vi "メイン.vi"() -> (2 "測定周期/ms":dbl, 3 "値転記用配列":T2[](array[typedef]))   [LabVIEW 2021] (continued)
        n1474 = local read "メイン設定_設定 6"() -> (w3404:T2)
        n1475 = Bundle By Name(cluster=w3404, "実測値(MAX)"=w3400, "実測値(MIN)"=w3400) -> (w3403:T2)
        n1476 = local write "メイン設定_設定 6"(w3403) -> ()
        n1477 = global write "測定値MAXMIN_G.vi" "測定値MAX/MINグローバル"(string[][] []) -> ()
      }
      frame "値7クリア" {
        w3405 = ""
        # "測定値MAX/MINグローバルの値を初期化する"
        # "②"
        # "①"
        # "複製したら変更する項目\n①②\nローカル変数\n\n変更のみでOK"
        # "項目別の値のクリアの為、項目配列の分だけ作成する"
        n1478 = local read "メイン設定_設定 7"() -> (w3409:T2)
        n1479 = Bundle By Name(cluster=w3409, "実測値(MAX)"=w3405, "実測値(MIN)"=w3405) -> (w3408:T2)
        n1480 = local write "メイン設定_設定 7"(w3408) -> ()
        n1481 = global write "測定値MAXMIN_G.vi" "測定値MAX/MINグローバル"(string[][] []) -> ()
      }
      frame "値8クリア" {
        w3410 = ""
        # "測定値MAX/MINグローバルの値を初期化する"
        # "②"
        # "①"
        # "複製したら変更する項目\n①②\nローカル変数\n\n変更のみでOK"
        # "項目別の値のクリアの為、項目配列の分だけ作成する"
        n1482 = local read "メイン設定_設定 8"() -> (w3414:T2)
        n1483 = Bundle By Name(cluster=w3414, "実測値(MAX)"=w3410, "実測値(MIN)"=w3410) -> (w3413:T2)
        n1484 = local write "メイン設定_設定 8"(w3413) -> ()
        n1485 = global write "測定値MAXMIN_G.vi" "測定値MAX/MINグローバル"(string[][] []) -> ()
      }
      frame "値9クリア" {
        w3415 = ""
        # "測定値MAX/MINグローバルの値を初期化する"
        # "②"
        # "①"
        # "複製したら変更する項目\n①②\nローカル変数\n\n変更のみでOK"
        # "項目別の値のクリアの為、項目配列の分だけ作成する"
        n1486 = local read "メイン設定_設定 9"() -> (w3419:T2)
        n1487 = Bundle By Name(cluster=w3419, "実測値(MAX)"=w3415, "実測値(MIN)"=w3415) -> (w3418:T2)
        n1488 = local write "メイン設定_設定 9"(w3418) -> ()
        n1489 = global write "測定値MAXMIN_G.vi" "測定値MAX/MINグローバル"(string[][] []) -> ()
      }
      frame "値10クリア" {
        w3420 = ""
        # "測定値MAX/MINグローバルの値を初期化する"
        # "②"
        # "①"
        # "複製したら変更する項目\n①②\nローカル変数\n\n変更のみでOK"
        # "項目別の値のクリアの為、項目配列の分だけ作成する"
        n1490 = local read "メイン設定_設定 10"() -> (w3424:T2)
        n1491 = Bundle By Name(cluster=w3424, "実測値(MAX)"=w3420, "実測値(MIN)"=w3420) -> (w3423:T2)
        n1492 = local write "メイン設定_設定 10"(w3423) -> ()
        n1493 = global write "測定値MAXMIN_G.vi" "測定値MAX/MINグローバル"(string[][] []) -> ()
      }
      frame "値11クリア" {
        w3425 = ""
        # "測定値MAX/MINグローバルの値を初期化する"
        # "②"
        # "①"
        # "複製したら変更する項目\n①②\nローカル変数\n\n変更のみでOK"
        # "項目別の値のクリアの為、項目配列の分だけ作成する"
        n1494 = local read "メイン設定_設定 11"() -> (w3429:T2)
        n1495 = Bundle By Name(cluster=w3429, "実測値(MAX)"=w3425, "実測値(MIN)"=w3425) -> (w3428:T2)
        n1496 = local write "メイン設定_設定 11"(w3428) -> ()
        n1497 = global write "測定値MAXMIN_G.vi" "測定値MAX/MINグローバル"(string[][] []) -> ()
      }
      frame "値12クリア" {
        w3430 = ""
        # "測定値MAX/MINグローバルの値を初期化する"
        # "②"
        # "①"
        # "複製したら変更する項目\n①②\nローカル変数\n\n変更のみでOK"
        # "項目別の値のクリアの為、項目配列の分だけ作成する"
        n1498 = local read "メイン設定_設定 12"() -> (w3434:T2)
        n1499 = Bundle By Name(cluster=w3434, "実測値(MAX)"=w3430, "実測値(MIN)"=w3430) -> (w3433:T2)
        n1500 = local write "メイン設定_設定 12"(w3433) -> ()
        n1501 = global write "測定値MAXMIN_G.vi" "測定値MAX/MINグローバル"(string[][] []) -> ()
      }
      frame "測定1" {
        # "項目別のボタンで測定を行う為、項目分必要"
        n1502 = local read "測定旧値 1"() -> (w3437:bool)
        n1503 = case shown="FALSE" w3437 {
          tunnel: w3435 -> [w3440 w3703]
          tunnel: [w3439 w3703] -> w3436
          frame False {
            n1504 = flat-sequence {
              tunnel: w3440 -> [w3450]
              tunnel: [w3441] -> w3438
              tunnel: [w3688] -> w3439
              tunnel: w3438 -> [w3688]
              frame #0 {
                # "※複製コピー時変更する項目\n①②\nローカル変数\n\n入れ子のケースストラクチャ\"2\"を複製\n\n0～数だけ変更する\n③④⑤\nローカル変数\n\n※AB\n行番号の変更をする必要がある\n\n--------------------------------\nこの後イベントストラクチャ複製する\n--------------------------------\nイベントストラクチャ複製後\n\n⑦⑧\nローカル変数\n⑨\n装飾体の位置設定\n-51は固定\n前ケースの数値+72\n⑩\n測定新値リセット用\nのボタンが複製されているので、\nフロントパネルを整理する\n⑪\nプロパティノード\nボタンの無効解除クリア以外全てのボタン対象"
                # "実測完了\n1)測定モードが単発・連続、多点かで転記する配列を変える\n2)値転記用配列へ転記\n\nここからゲージ分を繰り返す必要がある\n\n3)配列0を取り出す\n4)配列0のポートNoを取り出す\n5)メイン測定_設定配列(測定1の対象配列)のポートNoと比較\n6)同じだったら処理をする。違ったら何もしない\n7)同じだったら配列0のメインON/OFF_設定1の使用ON/OFFがTrueかFalseか\nFlaseだったら前回値転記用配列から前回の値をメイン設定_設定へ転記\nTrueだったらメイン設定_設定の測定モードから\n0単発、1連続、3多点\nの処理を行う\n8)測定値をメイン設定_設定へ転記したら、前回転記用配列へ転記する"
                # "グループNO(表示上はポートNo)が同じだったら値を転記する\n\n測定した配列のグループNOと値転記用配列の他の指標グループNOを比較する\n＝だったら、対象の配列のON/OFFボタンがTrueか確認し、\nTrueだったら、測定モードによって、値かMAX、MINの数値を転記する\n\nグループNOが同じでなければ、転記しない(何もしない)"
                # "まず値転記用配列に測定の値を転記"
                # "設定項目の値へ値転記用配列から転記\n測定モードによって転記の値をMAXのみするか\nMAXとMINにするか分ける"
                # "実測定画面vi動作"
                n1505 = local read "メイン設定_設定 1"() -> (w3447:T2)
                n1506 = local read "測定周期/ms"() -> (w3448:dbl)
                n1507 = local read "測定新値 1"() -> (→"測定新値\nリセット用 1":bool)
                n1508 = Unbundle By Name(w3447) -> ("測定モード"=w3446:u16)
                n1509 = call "実測定画面.vi"("実測設定項目配列_\nメインからの転記"=w3450, "測定周期/ms_制御器"=w3448) -> ("実測設定項目配列_\nゲージIOへ転記用"=w3445:T2[], "実測設定項目配列_\n多点測定メイン転記用"=w3444:T2[])  [unwired: 11 in, 1 out]
                n1510 = case shown="2" w3446 {
                  tunnel: w3445 -> [w3457 w3458 _]
                  tunnel: [w3457 w3458 w3459] -> w3442
                  tunnel: w3444 -> [_ _ w3459]
                  frame 0, Default {
                  }
                  frame 1 {
                  }
                  frame 2 {
                  }
                }
                n1511 = for {
                  N: 32 -> [_]
                  tunnel: w3442 -> [w3466]
                  i -> [w3461]
                  # "32回分"
                  # "比較する固定GNO"
                  n1512 = local read "メイン設定_設定 1"() -> (w3460:T2)
                  n1513 = Index Array(array=w3466, index=w3461) -> (element=w3465:T2)
                  n1514 = Unbundle By Name(w3465) -> ("ポートNo."=w3463:dbl)
                  n1515 = Unbundle By Name(w3460) -> ("ポートNo."=w3464:dbl)
                  n1516 = Equal?(x=w3464, y=w3463) -> (x = y?=w3462:bool)
                  n1517 = case shown="TRUE" w3462 {
                    tunnel: w3465 -> [_ w3468]
                    tunnel: w3461 -> [_ w3467]
                    frame False {
                    }
                    frame True {
                      n1518 = case shown="0, デフォルト" w3467 {
                        tunnel: w3468 -> [w3484 w3502 w3520 w3538 w3556 w3574 w3592 w3610 w3628 w3646 w3664 w3682]
                        tunnel: w3467 -> [w3483 w3501 w3519 w3537 w3555 w3573 w3591 w3609 w3627 w3645 w3663 w3681]
                        frame 0, Default {
                          w3474 = 2
                          # "B"
                          # "A"
                          # "csv作成の為表へクラスタ(実測値)書き込み"
                          # "⑤"
                          # "③"
                          # "④"
                          n1519 = local read "メインON/OFF_\n設定 1"() -> (w3485:T1)
                          n1520 = Unbundle By Name(w3485) -> ("使用ON/OFF"=w3481:bool)
                          n1521 = control-ref of="前回値転記用配列"() -> (w3479:refnum<vi>)
                          n1522 = local read "メイン設定_設定 1"() -> (w3486:T2)
                          n1523 = call "メイン_測定値配列_CSV転記サブ.vi"("メイン設定_設定入力"=w3486, "ループ反復数値入力"=w3483, "実測設定項目"=w3484, "使用ON/OFF"=w3481, "前回値転記用配列"=w3479) -> ("ループ反復数値出力"=w3482:i32, "メイン設定_設定出力"=w3480:T2)  [unwired: 5 in]
                          n1524 = local write "メイン設定_設定 1"(w3480) -> ()
                          n1525 = Add(x=2, y=w3482) -> (x+y=w3475:i32)
                          n1526 = Add(x=w3482, y=3) -> (x+y=w3473:i32)
                          n1527 = local read "csv作成表"() -> (w3469:string[][])
                          n1528 = Unbundle By Name(w3480) -> ("実測値(MAX)"=w3476:string, "実測値(MIN)"=w3477:string)
                          n1529 = Replace Array Subset(array=w3469, new element #1=w3476, index (row) #1=w3474, index (col) #1=w3475, new element #2=w3477, index (row) #2=w3474, index (col) #2=w3473) -> (w3471:string[][])
                          n1530 = Select(t=w3471, s=w3481, f=w3469) -> (s? t:f=w3472:string[][])
                          n1531 = local write "csv作成表"(w3472) -> ()
                        }
                        frame 1 {
                          w3492 = 2
                          # "B"
                          # "A"
                          # "csv作成の為表へクラスタ(実測値)書き込み"
                          # "⑤"
                          # "③"
                          # "④"
                          n1532 = local read "メインON/OFF_\n設定 2"() -> (w3503:T1)
                          n1533 = Unbundle By Name(w3503) -> ("使用ON/OFF"=w3499:bool)
                          n1534 = control-ref of="前回値転記用配列"() -> (w3497:refnum<vi>)
                          n1535 = local read "メイン設定_設定 2"() -> (w3504:T2)
                          n1536 = call "メイン_測定値配列_CSV転記サブ.vi"("メイン設定_設定入力"=w3504, "ループ反復数値入力"=w3501, "実測設定項目"=w3502, "使用ON/OFF"=w3499, "前回値転記用配列"=w3497) -> ("ループ反復数値出力"=w3500:i32, "メイン設定_設定出力"=w3498:T2)  [unwired: 5 in]
                          n1537 = local write "メイン設定_設定 2"(w3498) -> ()
                          n1538 = Add(x=3, y=w3500) -> (x+y=w3493:i32)
                          n1539 = Add(x=w3500, y=4) -> (x+y=w3491:i32)
                          n1540 = local read "csv作成表"() -> (w3487:string[][])
                          n1541 = Unbundle By Name(w3498) -> ("実測値(MAX)"=w3494:string, "実測値(MIN)"=w3495:string)
                          n1542 = Replace Array Subset(array=w3487, new element #1=w3494, index (row) #1=w3492, index (col) #1=w3493, new element #2=w3495, index (row) #2=w3492, index (col) #2=w3491) -> (w3489:string[][])
                          n1543 = Select(t=w3489, s=w3499, f=w3487) -> (s? t:f=w3490:string[][])
                          n1544 = local write "csv作成表"(w3490) -> ()
                        }
                        frame 2 {
                          w3510 = 2
                          # "B"
                          # "A"
                          # "csv作成の為表へクラスタ(実測値)書き込み"
                          # "⑤"
                          # "③"
                          # "④"
                          n1545 = local read "メインON/OFF_\n設定 3"() -> (w3521:T1)
                          n1546 = Unbundle By Name(w3521) -> ("使用ON/OFF"=w3517:bool)
                          n1547 = control-ref of="前回値転記用配列"() -> (w3515:refnum<vi>)
                          n1548 = local read "メイン設定_設定 3"() -> (w3522:T2)
                          n1549 = call "メイン_測定値配列_CSV転記サブ.vi"("メイン設定_設定入力"=w3522, "ループ反復数値入力"=w3519, "実測設定項目"=w3520, "使用ON/OFF"=w3517, "前回値転記用配列"=w3515) -> ("ループ反復数値出力"=w3518:i32, "メイン設定_設定出力"=w3516:T2)  [unwired: 5 in]
                          n1550 = local write "メイン設定_設定 3"(w3516) -> ()
                          n1551 = Add(x=4, y=w3518) -> (x+y=w3511:i32)
                          n1552 = Add(x=w3518, y=5) -> (x+y=w3509:i32)
                          n1553 = local read "csv作成表"() -> (w3505:string[][])
                          n1554 = Unbundle By Name(w3516) -> ("実測値(MAX)"=w3512:string, "実測値(MIN)"=w3513:string)
                          n1555 = Replace Array Subset(array=w3505, new element #1=w3512, index (row) #1=w3510, index (col) #1=w3511, new element #2=w3513, index (row) #2=w3510, index (col) #2=w3509) -> (w3507:string[][])
                          n1556 = Select(t=w3507, s=w3517, f=w3505) -> (s? t:f=w3508:string[][])
                          n1557 = local write "csv作成表"(w3508) -> ()
                        }
                        frame 3 {
                          w3528 = 2
                          # "B"
                          # "A"
                          # "csv作成の為表へクラスタ(実測値)書き込み"
                          # "⑤"
                          # "③"
                          # "④"
                          n1558 = local read "メインON/OFF_\n設定 4"() -> (w3539:T1)
                          n1559 = Unbundle By Name(w3539) -> ("使用ON/OFF"=w3535:bool)
                          n1560 = control-ref of="前回値転記用配列"() -> (w3533:refnum<vi>)
                          n1561 = local read "メイン設定_設定 4"() -> (w3540:T2)
                          n1562 = call "メイン_測定値配列_CSV転記サブ.vi"("メイン設定_設定入力"=w3540, "ループ反復数値入力"=w3537, "実測設定項目"=w3538, "使用ON/OFF"=w3535, "前回値転記用配列"=w3533) -> ("ループ反復数値出力"=w3536:i32, "メイン設定_設定出力"=w3534:T2)  [unwired: 5 in]
                          n1563 = local write "メイン設定_設定 4"(w3534) -> ()
                          n1564 = Add(x=5, y=w3536) -> (x+y=w3529:i32)
                          n1565 = Add(x=w3536, y=6) -> (x+y=w3527:i32)
                          n1566 = local read "csv作成表"() -> (w3523:string[][])
                          n1567 = Unbundle By Name(w3534) -> ("実測値(MAX)"=w3530:string, "実測値(MIN)"=w3531:string)
                          n1568 = Replace Array Subset(array=w3523, new element #1=w3530, index (row) #1=w3528, index (col) #1=w3529, new element #2=w3531, index (row) #2=w3528, index (col) #2=w3527) -> (w3525:string[][])
                          n1569 = Select(t=w3525, s=w3535, f=w3523) -> (s? t:f=w3526:string[][])
                          n1570 = local write "csv作成表"(w3526) -> ()
                        }
                        frame 4 {
                          w3546 = 2
                          # "B"
                          # "A"
                          # "csv作成の為表へクラスタ(実測値)書き込み"
                          # "⑤"
                          # "③"
                          # "④"
                          n1571 = local read "メインON/OFF_\n設定 5"() -> (w3557:T1)
                          n1572 = Unbundle By Name(w3557) -> ("使用ON/OFF"=w3553:bool)
                          n1573 = control-ref of="前回値転記用配列"() -> (w3551:refnum<vi>)
                          n1574 = local read "メイン設定_設定 5"() -> (w3558:T2)
                          n1575 = call "メイン_測定値配列_CSV転記サブ.vi"("メイン設定_設定入力"=w3558, "ループ反復数値入力"=w3555, "実測設定項目"=w3556, "使用ON/OFF"=w3553, "前回値転記用配列"=w3551) -> ("ループ反復数値出力"=w3554:i32, "メイン設定_設定出力"=w3552:T2)  [unwired: 5 in]
                          n1576 = local write "メイン設定_設定 5"(w3552) -> ()
                          n1577 = Add(x=6, y=w3554) -> (x+y=w3547:i32)
                          n1578 = Add(x=w3554, y=7) -> (x+y=w3545:i32)
                          n1579 = local read "csv作成表"() -> (w3541:string[][])
                          n1580 = Unbundle By Name(w3552) -> ("実測値(MAX)"=w3548:string, "実測値(MIN)"=w3549:string)
                          n1581 = Replace Array Subset(array=w3541, new element #1=w3548, index (row) #1=w3546, index (col) #1=w3547, new element #2=w3549, index (row) #2=w3546, index (col) #2=w3545) -> (w3543:string[][])
                          n1582 = Select(t=w3543, s=w3553, f=w3541) -> (s? t:f=w3544:string[][])
                          n1583 = local write "csv作成表"(w3544) -> ()
                        }
                        frame 5 {
                          w3564 = 2
                          # "B"
                          # "A"
                          # "csv作成の為表へクラスタ(実測値)書き込み"
                          # "⑤"
                          # "③"
                          # "④"
                          n1584 = local read "メインON/OFF_\n設定 6"() -> (w3575:T1)
                          n1585 = Unbundle By Name(w3575) -> ("使用ON/OFF"=w3571:bool)
                          n1586 = control-ref of="前回値転記用配列"() -> (w3569:refnum<vi>)
                          n1587 = local read "メイン設定_設定 6"() -> (w3576:T2)
                          n1588 = call "メイン_測定値配列_CSV転記サブ.vi"("メイン設定_設定入力"=w3576, "ループ反復数値入力"=w3573, "実測設定項目"=w3574, "使用ON/OFF"=w3571, "前回値転記用配列"=w3569) -> ("ループ反復数値出力"=w3572:i32, "メイン設定_設定出力"=w3570:T2)  [unwired: 5 in]
                          n1589 = local write "メイン設定_設定 6"(w3570) -> ()
                          n1590 = Add(x=7, y=w3572) -> (x+y=w3565:i32)
                          n1591 = Add(x=w3572, y=8) -> (x+y=w3563:i32)
                          n1592 = local read "csv作成表"() -> (w3559:string[][])
                          n1593 = Unbundle By Name(w3570) -> ("実測値(MAX)"=w3566:string, "実測値(MIN)"=w3567:string)
                          n1594 = Replace Array Subset(array=w3559, new element #1=w3566, index (row) #1=w3564, index (col) #1=w3565, new element #2=w3567, index (row) #2=w3564, index (col) #2=w3563) -> (w3561:string[][])
                          n1595 = Select(t=w3561, s=w3571, f=w3559) -> (s? t:f=w3562:string[][])
                          n1596 = local write "csv作成表"(w3562) -> ()
                        }
                        frame 6 {
                          w3582 = 2
                          # "B"
                          # "A"
                          # "csv作成の為表へクラスタ(実測値)書き込み"
                          # "⑤"
                          # "③"
                          # "④"
                          n1597 = local read "メインON/OFF_\n設定 7"() -> (w3593:T1)
                          n1598 = Unbundle By Name(w3593) -> ("使用ON/OFF"=w3589:bool)
                          n1599 = control-ref of="前回値転記用配列"() -> (w3587:refnum<vi>)
                          n1600 = local read "メイン設定_設定 7"() -> (w3594:T2)
                          n1601 = call "メイン_測定値配列_CSV転記サブ.vi"("メイン設定_設定入力"=w3594, "ループ反復数値入力"=w3591, "実測設定項目"=w3592, "使用ON/OFF"=w3589, "前回値転記用配列"=w3587) -> ("ループ反復数値出力"=w3590:i32, "メイン設定_設定出力"=w3588:T2)  [unwired: 5 in]
                          n1602 = local write "メイン設定_設定 7"(w3588) -> ()
                          n1603 = Add(x=8, y=w3590) -> (x+y=w3583:i32)
                          n1604 = Add(x=w3590, y=9) -> (x+y=w3581:i32)
                          n1605 = local read "csv作成表"() -> (w3577:string[][])
                          n1606 = Unbundle By Name(w3588) -> ("実測値(MAX)"=w3584:string, "実測値(MIN)"=w3585:string)
                          n1607 = Replace Array Subset(array=w3577, new element #1=w3584, index (row) #1=w3582, index (col) #1=w3583, new element #2=w3585, index (row) #2=w3582, index (col) #2=w3581) -> (w3579:string[][])
                          n1608 = Select(t=w3579, s=w3589, f=w3577) -> (s? t:f=w3580:string[][])
                          n1609 = local write "csv作成表"(w3580) -> ()
                        }
                        frame 7 {
                          w3600 = 2
                          # "B"
                          # "A"
                          # "csv作成の為表へクラスタ(実測値)書き込み"
                          # "⑤"
                          # "③"
                          # "④"
                          n1610 = local read "メインON/OFF_\n設定 8"() -> (w3611:T1)
                          n1611 = Unbundle By Name(w3611) -> ("使用ON/OFF"=w3607:bool)
                          n1612 = control-ref of="前回値転記用配列"() -> (w3605:refnum<vi>)
                          n1613 = local read "メイン設定_設定 8"() -> (w3612:T2)
                          n1614 = call "メイン_測定値配列_CSV転記サブ.vi"("メイン設定_設定入力"=w3612, "ループ反復数値入力"=w3609, "実測設定項目"=w3610, "使用ON/OFF"=w3607, "前回値転記用配列"=w3605) -> ("ループ反復数値出力"=w3608:i32, "メイン設定_設定出力"=w3606:T2)  [unwired: 5 in]
                          n1615 = local write "メイン設定_設定 8"(w3606) -> ()
                          n1616 = Add(x=9, y=w3608) -> (x+y=w3601:i32)
                          n1617 = Add(x=w3608, y=10) -> (x+y=w3599:i32)
                          n1618 = local read "csv作成表"() -> (w3595:string[][])
                          n1619 = Unbundle By Name(w3606) -> ("実測値(MAX)"=w3602:string, "実測値(MIN)"=w3603:string)
                          n1620 = Replace Array Subset(array=w3595, new element #1=w3602, index (row) #1=w3600, index (col) #1=w3601, new element #2=w3603, index (row) #2=w3600, index (col) #2=w3599) -> (w3597:string[][])
                          n1621 = Select(t=w3597, s=w3607, f=w3595) -> (s? t:f=w3598:string[][])
                          n1622 = local write "csv作成表"(w3598) -> ()
                        }
                        frame 8 {
                          w3618 = 2
                          # "B"
                          # "A"
                          # "csv作成の為表へクラスタ(実測値)書き込み"
                          # "⑤"
                          # "③"
                          # "④"
                          n1623 = local read "メインON/OFF_\n設定 9"() -> (w3629:T1)
                          n1624 = Unbundle By Name(w3629) -> ("使用ON/OFF"=w3625:bool)
                          n1625 = control-ref of="前回値転記用配列"() -> (w3623:refnum<vi>)
                          n1626 = local read "メイン設定_設定 9"() -> (w3630:T2)
                          n1627 = call "メイン_測定値配列_CSV転記サブ.vi"("メイン設定_設定入力"=w3630, "ループ反復数値入力"=w3627, "実測設定項目"=w3628, "使用ON/OFF"=w3625, "前回値転記用配列"=w3623) -> ("ループ反復数値出力"=w3626:i32, "メイン設定_設定出力"=w3624:T2)  [unwired: 5 in]
                          n1628 = local write "メイン設定_設定 9"(w3624) -> ()
                          n1629 = Add(x=10, y=w3626) -> (x+y=w3619:i32)
                          n1630 = Add(x=w3626, y=11) -> (x+y=w3617:i32)
                          n1631 = local read "csv作成表"() -> (w3613:string[][])
                          n1632 = Unbundle By Name(w3624) -> ("実測値(MAX)"=w3620:string, "実測値(MIN)"=w3621:string)
                          n1633 = Replace Array Subset(array=w3613, new element #1=w3620, index (row) #1=w3618, index (col) #1=w3619, new element #2=w3621, index (row) #2=w3618, index (col) #2=w3617) -> (w3615:string[][])
                          n1634 = Select(t=w3615, s=w3625, f=w3613) -> (s? t:f=w3616:string[][])
                          n1635 = local write "csv作成表"(w3616) -> ()
                        }
                        frame 9 {
                          w3636 = 2
                          # "B"
                          # "A"
                          # "csv作成の為表へクラスタ(実測値)書き込み"
                          # "⑤"
                          # "③"
                          # "④"
                          n1636 = local read "メインON/OFF_\n設定 10"() -> (w3647:T1)
                          n1637 = Unbundle By Name(w3647) -> ("使用ON/OFF"=w3643:bool)
                          n1638 = control-ref of="前回値転記用配列"() -> (w3641:refnum<vi>)
                          n1639 = local read "メイン設定_設定 10"() -> (w3648:T2)
                          n1640 = call "メイン_測定値配列_CSV転記サブ.vi"("メイン設定_設定入力"=w3648, "ループ反復数値入力"=w3645, "実測設定項目"=w3646, "使用ON/OFF"=w3643, "前回値転記用配列"=w3641) -> ("ループ反復数値出力"=w3644:i32, "メイン設定_設定出力"=w3642:T2)  [unwired: 5 in]
                          n1641 = local write "メイン設定_設定 10"(w3642) -> ()
                          n1642 = Add(x=11, y=w3644) -> (x+y=w3637:i32)
                          n1643 = Add(x=w3644, y=12) -> (x+y=w3635:i32)
                          n1644 = local read "csv作成表"() -> (w3631:string[][])
                          n1645 = Unbundle By Name(w3642) -> ("実測値(MAX)"=w3638:string, "実測値(MIN)"=w3639:string)
                          n1646 = Replace Array Subset(array=w3631, new element #1=w3638, index (row) #1=w3636, index (col) #1=w3637, new element #2=w3639, index (row) #2=w3636, index (col) #2=w3635) -> (w3633:string[][])
                          n1647 = Select(t=w3633, s=w3643, f=w3631) -> (s? t:f=w3634:string[][])
                          n1648 = local write "csv作成表"(w3634) -> ()
                        }
                        frame 10 {
                          w3654 = 2
                          # "B"
                          # "A"
                          # "csv作成の為表へクラスタ(実測値)書き込み"
                          # "⑤"
                          # "③"
                          # "④"
                          n1649 = local read "メインON/OFF_\n設定 11"() -> (w3665:T1)
                          n1650 = Unbundle By Name(w3665) -> ("使用ON/OFF"=w3661:bool)
                          n1651 = control-ref of="前回値転記用配列"() -> (w3659:refnum<vi>)
                          n1652 = local read "メイン設定_設定 11"() -> (w3666:T2)
                          n1653 = call "メイン_測定値配列_CSV転記サブ.vi"("メイン設定_設定入力"=w3666, "ループ反復数値入力"=w3663, "実測設定項目"=w3664, "使用ON/OFF"=w3661, "前回値転記用配列"=w3659) -> ("ループ反復数値出力"=w3662:i32, "メイン設定_設定出力"=w3660:T2)  [unwired: 5 in]
                          n1654 = local write "メイン設定_設定 11"(w3660) -> ()
                          n1655 = Add(x=12, y=w3662) -> (x+y=w3655:i32)
                          n1656 = Add(x=w3662, y=13) -> (x+y=w3653:i32)
                          n1657 = local read "csv作成表"() -> (w3649:string[][])
                          n1658 = Unbundle By Name(w3660) -> ("実測値(MAX)"=w3656:string, "実測値(MIN)"=w3657:string)
                          n1659 = Replace Array Subset(array=w3649, new element #1=w3656, index (row) #1=w3654, index (col) #1=w3655, new element #2=w3657, index (row) #2=w3654, index (col) #2=w3653) -> (w3651:string[][])
                          n1660 = Select(t=w3651, s=w3661, f=w3649) -> (s? t:f=w3652:string[][])
                          n1661 = local write "csv作成表"(w3652) -> ()
                        }
                        frame 11 {
                          w3672 = 2
                          # "B"
                          # "A"
                          # "csv作成の為表へクラスタ(実測値)書き込み"
                          # "⑤"
                          # "③"
                          # "④"
                          n1662 = local read "メインON/OFF_\n設定 12"() -> (w3683:T1)
                          n1663 = Unbundle By Name(w3683) -> ("使用ON/OFF"=w3679:bool)
                          n1664 = control-ref of="前回値転記用配列"() -> (w3677:refnum<vi>)
                          n1665 = local read "メイン設定_設定 12"() -> (w3684:T2)
                          n1666 = call "メイン_測定値配列_CSV転記サブ.vi"("メイン設定_設定入力"=w3684, "ループ反復数値入力"=w3681, "実測設定項目"=w3682, "使用ON/OFF"=w3679, "前回値転記用配列"=w3677) -> ("ループ反復数値出力"=w3680:i32, "メイン設定_設定出力"=w3678:T2)  [unwired: 5 in]
                          n1667 = local write "メイン設定_設定 12"(w3678) -> ()
                          n1668 = Add(x=13, y=w3680) -> (x+y=w3673:i32)
                          n1669 = Add(x=w3680, y=14) -> (x+y=w3671:i32)
                          n1670 = local read "csv作成表"() -> (w3667:string[][])
                          n1671 = Unbundle By Name(w3678) -> ("実測値(MAX)"=w3674:string, "実測値(MIN)"=w3675:string)
                          n1672 = Replace Array Subset(array=w3667, new element #1=w3674, index (row) #1=w3672, index (col) #1=w3673, new element #2=w3675, index (row) #2=w3672, index (col) #2=w3671) -> (w3669:string[][])
                          n1673 = Select(t=w3669, s=w3679, f=w3667) -> (s? t:f=w3670:string[][])
                          n1674 = local write "csv作成表"(w3670) -> ()
                        }
                      }
                    }
                  }
                }
                n1675 = local write "値転記用配列"(w3442) -> ()
                n1676 = flat-sequence {
                  tunnel: w3442 -> [w3456]
                  tunnel: [w3456] -> w3441
                  frame #0 {
                    w3451 = T9 {"Horizontal"=-51, "Vertical"=0} ("座標 1")
                    n1677 = control-ref of="このVI"() -> (w3455:refnum<vi>)
                    n1678 = property on="ペーン 2" class="Pane"("Origin"=w3451) -> ()  [unwired: 2 in, 2 out]
                    n1679 = property on="ペーン 2" class="Pane"("Origin"=w3451) -> ()  [unwired: 2 in, 2 out]
                    n1680 = control-ref of="このVI"() -> (w3453:refnum<vi>)
                    n1681 = Unbundle(w3451) -> ("Vertical"=w3454:i16)  [unwired: 1 out]
                    n1682 = Unbundle(w3451) -> ("Vertical"=w3452:i16)  [unwired: 1 out]
                    n1683 = call "メイン_装飾移動サブ.vi"("Y軸座標入力"=w3454, "VI入力"=w3455) -> ()  [unwired: 10 in]
                    n1684 = call "メイン_装飾枠移動サブ.vi"("Y軸座標入力"=w3452, "VI入力"=w3453) -> ()  [unwired: 10 in]
                  }
                }
              }
              frame #1 {
                w3686 = T8."Enabled" ("無効")
                n1685 = for {
                  N: 12 -> [_]
                  tunnel: w3686 -> [w3689]
                  i -> [w3690]
                  n1686 = case shown="0, デフォルト" w3690 {
                    tunnel: w3689 -> [w3691 w3692 w3693 w3694 w3695 w3696 w3697 w3698 w3699 w3700 w3701 w3702]
                    frame 0, Default {
                      n1687 = property on="メイン測定ボタン_単発 1" class="Bool (指定)"("DisabledEnum"=w3691) -> ()  [unwired: 2 in, 2 out]
                      n1688 = property on="メイン測定ボタン_連続 1" class="Bool (指定)"("DisabledEnum"=w3691) -> ()  [unwired: 2 in, 2 out]
                    }
                    frame 1 {
                      n1689 = property on="メイン測定ボタン_単発 2" class="Bool (指定)"("DisabledEnum"=w3692) -> ()  [unwired: 2 in, 2 out]
                      n1690 = property on="メイン測定ボタン_連続 2" class="Bool (指定)"("DisabledEnum"=w3692) -> ()  [unwired: 2 in, 2 out]
                    }
                    frame 2 {
                      n1691 = property on="メイン測定ボタン_単発 3" class="Bool (指定)"("DisabledEnum"=w3693) -> ()  [unwired: 2 in, 2 out]
                      n1692 = property on="メイン測定ボタン_連続 3" class="Bool (指定)"("DisabledEnum"=w3693) -> ()  [unwired: 2 in, 2 out]
                    }
                    frame 3 {
                      n1693 = property on="メイン測定ボタン_単発 4" class="Bool (指定)"("DisabledEnum"=w3694) -> ()  [unwired: 2 in, 2 out]
                      n1694 = property on="メイン測定ボタン_連続 4" class="Bool (指定)"("DisabledEnum"=w3694) -> ()  [unwired: 2 in, 2 out]
                    }
                    frame 4 {
                      n1695 = property on="メイン測定ボタン_単発 5" class="Bool (指定)"("DisabledEnum"=w3695) -> ()  [unwired: 2 in, 2 out]
                      n1696 = property on="メイン測定ボタン_連続 5" class="Bool (指定)"("DisabledEnum"=w3695) -> ()  [unwired: 2 in, 2 out]
                    }
                    frame 5 {
                      n1697 = property on="メイン測定ボタン_連続 6" class="Bool (指定)"("DisabledEnum"=w3696) -> ()  [unwired: 2 in, 2 out]
                      n1698 = property on="メイン測定ボタン_単発 6" class="Bool (指定)"("DisabledEnum"=w3696) -> ()  [unwired: 2 in, 2 out]
                    }
                    frame 6 {
                      n1699 = property on="メイン測定ボタン_連続 7" class="Bool (指定)"("DisabledEnum"=w3697) -> ()  [unwired: 2 in, 2 out]
                      n1700 = property on="メイン測定ボタン_単発 7" class="Bool (指定)"("DisabledEnum"=w3697) -> ()  [unwired: 2 in, 2 out]
                    }
                    frame 7 {
                      n1701 = property on="メイン測定ボタン_単発 8" class="Bool (指定)"("DisabledEnum"=w3698) -> ()  [unwired: 2 in, 2 out]
                      n1702 = property on="メイン測定ボタン_連続 8" class="Bool (指定)"("DisabledEnum"=w3698) -> ()  [unwired: 2 in, 2 out]
                    }
                    frame 8 {
                      n1703 = property on="メイン測定ボタン_単発 9" class="Bool (指定)"("DisabledEnum"=w3699) -> ()  [unwired: 2 in, 2 out]
                      n1704 = property on="メイン測定ボタン_連続 9" class="Bool (指定)"("DisabledEnum"=w3699) -> ()  [unwired: 2 in, 2 out]
                    }
                    frame 9 {
                      n1705 = property on="メイン測定ボタン_単発 10" class="Bool (指定)"("DisabledEnum"=w3700) -> ()  [unwired: 2 in, 2 out]
                      n1706 = property on="メイン測定ボタン_連続 10" class="Bool (指定)"("DisabledEnum"=w3700) -> ()  [unwired: 2 in, 2 out]
                    }
                    frame 10 {
                      n1707 = property on="メイン測定ボタン_単発 11" class="Bool (指定)"("DisabledEnum"=w3701) -> ()  [unwired: 2 in, 2 out]
                      n1708 = property on="メイン測定ボタン_連続 11" class="Bool (指定)"("DisabledEnum"=w3701) -> ()  [unwired: 2 in, 2 out]
                    }
                    frame 11 {
                      n1709 = property on="メイン測定ボタン_連続 12" class="Bool (指定)"("DisabledEnum"=w3702) -> ()  [unwired: 2 in, 2 out]
                      n1710 = property on="メイン測定ボタン_単発 12" class="Bool (指定)"("DisabledEnum"=w3702) -> ()  [unwired: 2 in, 2 out]
                    }
                  }
                }
                n1711 = local write "測定新値\nリセット用 1"(TRUE) -> ()
                n1712 = property on="TOPページへ" class="Bool"("DisabledEnum"=w3686) -> ()  [unwired: 2 in, 2 out]
                n1713 = property on="保存して終了" class="Bool"("DisabledEnum"=w3686) -> ()  [unwired: 2 in, 2 out]
                n1714 = property on="保存せずに" class="Bool"("DisabledEnum"=w3686) -> ()  [unwired: 2 in, 2 out]
              }
            }
          }
          frame True {
          }
        }
      }
      frame "測定2" {
        # "⑦"
        # "項目別のボタンで測定を行う為、項目分必要"
        n1715 = local read "測定旧値 2"() -> (w3706:bool)
        n1716 = case shown="FALSE" w3706 {
          tunnel: w3704 -> [w3709 w3972]
          tunnel: [w3708 w3972] -> w3705
          frame False {
            n1717 = flat-sequence {
              tunnel: w3709 -> [w3719]
              tunnel: [w3710] -> w3707
              tunnel: [w3957] -> w3708
              tunnel: w3707 -> [w3957]
              frame #0 {
                # "※複製コピー時変更する項目\n①②\nローカル変数\n\n入れ子のケースストラクチャ\"2\"を複製\n\n0～数だけ変更する\n③④⑤\nローカル変数\n\n※AB\n行番号の変更をする必要がある\n\n--------------------------------\nこの後イベントストラクチャ複製する\n--------------------------------\nイベントストラクチャ複製後\n\n⑦⑧\nローカル変数\n⑨\n装飾体の位置設定\n-51は固定\n前ケースの数値+72\n⑩\n測定新値リセット用\nのボタンが複製されているので、\nフロントパネルを整理する\n⑪\nプロパティノード\nボタンの無効解除クリア以外全てのボタン対象"
                # "実測完了の簡易疑似コード\n\n1)測定モードが単発・連続、多点かで転記する配列を変える\n2)値転記用配列へ転記\n\nここからゲージ分を繰り返す必要がある\n\n3)配列0を取り出す\n4)配列0のポートNoを取り出す\n5)メイン測定_設定配列(測定1の対象配列)のポートNoと比較\n6)同じだったら処理をする。違ったら何もしない\n7)同じだったら配列0のメインON/OFF_設定1の使用ON/OFFがTrueかFalseか\nFlaseだったら前回値転記用配列から前回の値をメイン設定_設定へ転記\nTrueだったらメイン設定_設定の測定モードから\n0単発、1連続、3多点\nの処理を行う\n8)測定値をメイン設定_設定へ転記したら、前回転記用配列へ転記する"
                # "⑨"
                # "⑧"
                # "②"
                # "グループNO(表示上はポートNo)が同じだったら値を転記する\n\n測定した配列のグループNOと値転記用配列の他の指標グループNOを比較する\n＝だったら、対象の配列のON/OFFボタンがTrueか確認し、\nTrueだったら、測定モードによって、値かMAX、MINの数値を転記する\n\nグループNOが同じでなければ、転記しない(何もしない)"
                # "まず値転記用配列に測定の値を転記"
                # "実測定画面vi動作"
                n1718 = local read "メイン設定_設定 2"() -> (w3714:T2)
                n1719 = local read "測定新値 2"() -> (→"測定新値\nリセット用 2":bool)
                n1720 = local read "測定周期/ms"() -> (w3712:dbl)
                n1721 = Unbundle By Name(w3714) -> ("測定モード"=w3715:u16)
                n1722 = call "実測定画面.vi"("実測設定項目配列_\nメインからの転記"=w3719, "測定周期/ms_制御器"=w3712) -> ("実測設定項目配列_\nゲージIOへ転記用"=w3717:T2[], "実測設定項目配列_\n多点測定メイン転記用"=w3716:T2[])  [unwired: 11 in, 1 out]
                n1723 = case shown="0, デフォルト" w3715 {
                  tunnel: w3717 -> [w3726 w3727 _]
                  tunnel: [w3726 w3727 w3728] -> w3711
                  tunnel: w3716 -> [_ _ w3728]
                  frame 0, Default {
                  }
                  frame 1 {
                  }
                  frame 2 {
                  }
                }
                n1724 = for {
                  N: 32 -> [_]
                  tunnel: w3711 -> [w3735]
                  i -> [w3730]
                  # "①"
                  # "※複製コピーはこのケースで行う"
                  # "32回分"
                  # "比較する固定GNO"
                  n1725 = local read "メイン設定_設定 2"() -> (w3729:T2)
                  n1726 = Index Array(array=w3735, index=w3730) -> (element=w3734:T2)
                  n1727 = Unbundle By Name(w3729) -> ("ポートNo."=w3733:dbl)
                  n1728 = Unbundle By Name(w3734) -> ("ポートNo."=w3732:dbl)
                  n1729 = Equal?(x=w3733, y=w3732) -> (x = y?=w3731:bool)
                  n1730 = case shown="TRUE" w3731 {
                    tunnel: w3734 -> [_ w3737]
                    tunnel: w3730 -> [_ w3736]
                    frame False {
                    }
                    frame True {
                      n1731 = case shown="0, デフォルト" w3736 {
                        tunnel: w3737 -> [w3753 w3771 w3789 w3807 w3825 w3843 w3861 w3879 w3897 w3915 w3933 w3951]
                        tunnel: w3736 -> [w3752 w3770 w3788 w3806 w3824 w3842 w3860 w3878 w3896 w3914 w3932 w3950]
                        frame 0, Default {
                          w3743 = 2
                          # "B"
                          # "A"
                          # "csv作成の為表へクラスタ(実測値)書き込み"
                          # "⑤"
                          # "③"
                          # "④"
                          n1732 = local read "メインON/OFF_\n設定 1"() -> (w3754:T1)
                          n1733 = Unbundle By Name(w3754) -> ("使用ON/OFF"=w3750:bool)
                          n1734 = control-ref of="前回値転記用配列"() -> (w3748:refnum<vi>)
                          n1735 = local read "メイン設定_設定 1"() -> (w3755:T2)
                          n1736 = call "メイン_測定値配列_CSV転記サブ.vi"("メイン設定_設定入力"=w3755, "ループ反復数値入力"=w3752, "実測設定項目"=w3753, "使用ON/OFF"=w3750, "前回値転記用配列"=w3748) -> ("ループ反復数値出力"=w3751:i32, "メイン設定_設定出力"=w3749:T2)  [unwired: 5 in]
                          n1737 = local write "メイン設定_設定 1"(w3749) -> ()
                          n1738 = Add(x=2, y=w3751) -> (x+y=w3744:i32)
                          n1739 = Add(x=w3751, y=3) -> (x+y=w3742:i32)
                          n1740 = local read "csv作成表"() -> (w3738:string[][])
                          n1741 = Unbundle By Name(w3749) -> ("実測値(MAX)"=w3745:string, "実測値(MIN)"=w3746:string)
                          n1742 = Replace Array Subset(array=w3738, new element #1=w3745, index (row) #1=w3743, index (col) #1=w3744, new element #2=w3746, index (row) #2=w3743, index (col) #2=w3742) -> (w3740:string[][])
                          n1743 = Select(t=w3740, s=w3750, f=w3738) -> (s? t:f=w3741:string[][])
                          n1744 = local write "csv作成表"(w3741) -> ()
                        }
                        frame 1 {
                          w3761 = 2
                          # "B"
                          # "A"
                          # "csv作成の為表へクラスタ(実測値)書き込み"
                          # "⑤"
                          # "③"
                          # "④"
                          n1745 = local read "メインON/OFF_\n設定 2"() -> (w3772:T1)
                          n1746 = Unbundle By Name(w3772) -> ("使用ON/OFF"=w3768:bool)
                          n1747 = control-ref of="前回値転記用配列"() -> (w3766:refnum<vi>)
                          n1748 = local read "メイン設定_設定 2"() -> (w3773:T2)
                          n1749 = call "メイン_測定値配列_CSV転記サブ.vi"("メイン設定_設定入力"=w3773, "ループ反復数値入力"=w3770, "実測設定項目"=w3771, "使用ON/OFF"=w3768, "前回値転記用配列"=w3766) -> ("ループ反復数値出力"=w3769:i32, "メイン設定_設定出力"=w3767:T2)  [unwired: 5 in]
                          n1750 = local write "メイン設定_設定 2"(w3767) -> ()
                          n1751 = Add(x=3, y=w3769) -> (x+y=w3762:i32)
                          n1752 = Add(x=w3769, y=4) -> (x+y=w3760:i32)
                          n1753 = local read "csv作成表"() -> (w3756:string[][])
                          n1754 = Unbundle By Name(w3767) -> ("実測値(MAX)"=w3763:string, "実測値(MIN)"=w3764:string)
                          n1755 = Replace Array Subset(array=w3756, new element #1=w3763, index (row) #1=w3761, index (col) #1=w3762, new element #2=w3764, index (row) #2=w3761, index (col) #2=w3760) -> (w3758:string[][])
                          n1756 = Select(t=w3758, s=w3768, f=w3756) -> (s? t:f=w3759:string[][])
                          n1757 = local write "csv作成表"(w3759) -> ()
                        }
                        frame 2 {
                          w3779 = 2
                          # "B"
                          # "A"
                          # "csv作成の為表へクラスタ(実測値)書き込み"
                          # "⑤"
                          # "③"
                          # "④"
                          n1758 = local read "メインON/OFF_\n設定 3"() -> (w3790:T1)
                          n1759 = Unbundle By Name(w3790) -> ("使用ON/OFF"=w3786:bool)
                          n1760 = control-ref of="前回値転記用配列"() -> (w3784:refnum<vi>)
                          n1761 = local read "メイン設定_設定 3"() -> (w3791:T2)
                          n1762 = call "メイン_測定値配列_CSV転記サブ.vi"("メイン設定_設定入力"=w3791, "ループ反復数値入力"=w3788, "実測設定項目"=w3789, "使用ON/OFF"=w3786, "前回値転記用配列"=w3784) -> ("ループ反復数値出力"=w3787:i32, "メイン設定_設定出力"=w3785:T2)  [unwired: 5 in]
                          n1763 = local write "メイン設定_設定 3"(w3785) -> ()
                          n1764 = Add(x=4, y=w3787) -> (x+y=w3780:i32)
                          n1765 = Add(x=w3787, y=5) -> (x+y=w3778:i32)
                          n1766 = local read "csv作成表"() -> (w3774:string[][])
                          n1767 = Unbundle By Name(w3785) -> ("実測値(MAX)"=w3781:string, "実測値(MIN)"=w3782:string)
                          n1768 = Replace Array Subset(array=w3774, new element #1=w3781, index (row) #1=w3779, index (col) #1=w3780, new element #2=w3782, index (row) #2=w3779, index (col) #2=w3778) -> (w3776:string[][])
                          n1769 = Select(t=w3776, s=w3786, f=w3774) -> (s? t:f=w3777:string[][])
                          n1770 = local write "csv作成表"(w3777) -> ()
                        }
                        frame 3 {
                          w3797 = 2
                          # "B"
                          # "A"
                          # "csv作成の為表へクラスタ(実測値)書き込み"
                          # "⑤"
                          # "③"
                          # "④"
                          n1771 = local read "メインON/OFF_\n設定 4"() -> (w3808:T1)
                          n1772 = Unbundle By Name(w3808) -> ("使用ON/OFF"=w3804:bool)
                          n1773 = control-ref of="前回値転記用配列"() -> (w3802:refnum<vi>)
                          n1774 = local read "メイン設定_設定 4"() -> (w3809:T2)
                          n1775 = call "メイン_測定値配列_CSV転記サブ.vi"("メイン設定_設定入力"=w3809, "ループ反復数値入力"=w3806, "実測設定項目"=w3807, "使用ON/OFF"=w3804, "前回値転記用配列"=w3802) -> ("ループ反復数値出力"=w3805:i32, "メイン設定_設定出力"=w3803:T2)  [unwired: 5 in]
                          n1776 = local write "メイン設定_設定 4"(w3803) -> ()
                          n1777 = Add(x=5, y=w3805) -> (x+y=w3798:i32)
                          n1778 = Add(x=w3805, y=6) -> (x+y=w3796:i32)
                          n1779 = local read "csv作成表"() -> (w3792:string[][])
                          n1780 = Unbundle By Name(w3803) -> ("実測値(MAX)"=w3799:string, "実測値(MIN)"=w3800:string)
                          n1781 = Replace Array Subset(array=w3792, new element #1=w3799, index (row) #1=w3797, index (col) #1=w3798, new element #2=w3800, index (row) #2=w3797, index (col) #2=w3796) -> (w3794:string[][])
                          n1782 = Select(t=w3794, s=w3804, f=w3792) -> (s? t:f=w3795:string[][])
                          n1783 = local write "csv作成表"(w3795) -> ()
                        }
                        frame 4 {
                          w3815 = 2
                          # "B"
                          # "A"
                          # "csv作成の為表へクラスタ(実測値)書き込み"
                          # "⑤"
                          # "③"
                          # "④"
                          n1784 = local read "メインON/OFF_\n設定 5"() -> (w3826:T1)
                          n1785 = Unbundle By Name(w3826) -> ("使用ON/OFF"=w3822:bool)
                          n1786 = control-ref of="前回値転記用配列"() -> (w3820:refnum<vi>)
                          n1787 = local read "メイン設定_設定 5"() -> (w3827:T2)
                          n1788 = call "メイン_測定値配列_CSV転記サブ.vi"("メイン設定_設定入力"=w3827, "ループ反復数値入力"=w3824, "実測設定項目"=w3825, "使用ON/OFF"=w3822, "前回値転記用配列"=w3820) -> ("ループ反復数値出力"=w3823:i32, "メイン設定_設定出力"=w3821:T2)  [unwired: 5 in]
                          n1789 = local write "メイン設定_設定 5"(w3821) -> ()
                          n1790 = Add(x=6, y=w3823) -> (x+y=w3816:i32)
                          n1791 = Add(x=w3823, y=7) -> (x+y=w3814:i32)
                          n1792 = local read "csv作成表"() -> (w3810:string[][])
                          n1793 = Unbundle By Name(w3821) -> ("実測値(MAX)"=w3817:string, "実測値(MIN)"=w3818:string)
                          n1794 = Replace Array Subset(array=w3810, new element #1=w3817, index (row) #1=w3815, index (col) #1=w3816, new element #2=w3818, index (row) #2=w3815, index (col) #2=w3814) -> (w3812:string[][])
                          n1795 = Select(t=w3812, s=w3822, f=w3810) -> (s? t:f=w3813:string[][])
                          n1796 = local write "csv作成表"(w3813) -> ()
                        }
                        frame 5 {
                          w3833 = 2
                          # "B"
                          # "A"
                          # "csv作成の為表へクラスタ(実測値)書き込み"
                          # "⑤"
                          # "③"
                          # "④"
                          n1797 = local read "メインON/OFF_\n設定 6"() -> (w3844:T1)
                          n1798 = Unbundle By Name(w3844) -> ("使用ON/OFF"=w3840:bool)
                          n1799 = control-ref of="前回値転記用配列"() -> (w3838:refnum<vi>)
                          n1800 = local read "メイン設定_設定 6"() -> (w3845:T2)
                          n1801 = call "メイン_測定値配列_CSV転記サブ.vi"("メイン設定_設定入力"=w3845, "ループ反復数値入力"=w3842, "実測設定項目"=w3843, "使用ON/OFF"=w3840, "前回値転記用配列"=w3838) -> ("ループ反復数値出力"=w3841:i32, "メイン設定_設定出力"=w3839:T2)  [unwired: 5 in]
                          n1802 = local write "メイン設定_設定 6"(w3839) -> ()
                          n1803 = Add(x=7, y=w3841) -> (x+y=w3834:i32)
                          n1804 = Add(x=w3841, y=8) -> (x+y=w3832:i32)
                          n1805 = local read "csv作成表"() -> (w3828:string[][])
                          n1806 = Unbundle By Name(w3839) -> ("実測値(MAX)"=w3835:string, "実測値(MIN)"=w3836:string)
                          n1807 = Replace Array Subset(array=w3828, new element #1=w3835, index (row) #1=w3833, index (col) #1=w3834, new element #2=w3836, index (row) #2=w3833, index (col) #2=w3832) -> (w3830:string[][])
                          n1808 = Select(t=w3830, s=w3840, f=w3828) -> (s? t:f=w3831:string[][])
                          n1809 = local write "csv作成表"(w3831) -> ()
                        }
                        frame 6 {
                          w3851 = 2
                          # "B"
                          # "A"
                          # "csv作成の為表へクラスタ(実測値)書き込み"
                          # "⑤"
                          # "③"
                          # "④"
                          n1810 = local read "メインON/OFF_\n設定 7"() -> (w3862:T1)
                          n1811 = Unbundle By Name(w3862) -> ("使用ON/OFF"=w3858:bool)
                          n1812 = control-ref of="前回値転記用配列"() -> (w3856:refnum<vi>)
                          n1813 = local read "メイン設定_設定 7"() -> (w3863:T2)
                          n1814 = call "メイン_測定値配列_CSV転記サブ.vi"("メイン設定_設定入力"=w3863, "ループ反復数値入力"=w3860, "実測設定項目"=w3861, "使用ON/OFF"=w3858, "前回値転記用配列"=w3856) -> ("ループ反復数値出力"=w3859:i32, "メイン設定_設定出力"=w3857:T2)  [unwired: 5 in]
                          n1815 = local write "メイン設定_設定 7"(w3857) -> ()
                          n1816 = Add(x=8, y=w3859) -> (x+y=w3852:i32)
                          n1817 = Add(x=w3859, y=9) -> (x+y=w3850:i32)
                          n1818 = local read "csv作成表"() -> (w3846:string[][])
                          n1819 = Unbundle By Name(w3857) -> ("実測値(MAX)"=w3853:string, "実測値(MIN)"=w3854:string)
                          n1820 = Replace Array Subset(array=w3846, new element #1=w3853, index (row) #1=w3851, index (col) #1=w3852, new element #2=w3854, index (row) #2=w3851, index (col) #2=w3850) -> (w3848:string[][])
                          n1821 = Select(t=w3848, s=w3858, f=w3846) -> (s? t:f=w3849:string[][])
                          n1822 = local write "csv作成表"(w3849) -> ()
                        }
                        frame 7 {
                          w3869 = 2
                          # "B"
                          # "A"
                          # "csv作成の為表へクラスタ(実測値)書き込み"
                          # "⑤"
                          # "③"
                          # "④"
                          n1823 = local read "メインON/OFF_\n設定 8"() -> (w3880:T1)
                          n1824 = Unbundle By Name(w3880) -> ("使用ON/OFF"=w3876:bool)
                          n1825 = control-ref of="前回値転記用配列"() -> (w3874:refnum<vi>)
                          n1826 = local read "メイン設定_設定 8"() -> (w3881:T2)
                          n1827 = call "メイン_測定値配列_CSV転記サブ.vi"("メイン設定_設定入力"=w3881, "ループ反復数値入力"=w3878, "実測設定項目"=w3879, "使用ON/OFF"=w3876, "前回値転記用配列"=w3874) -> ("ループ反復数値出力"=w3877:i32, "メイン設定_設定出力"=w3875:T2)  [unwired: 5 in]
                          n1828 = local write "メイン設定_設定 8"(w3875) -> ()
                          n1829 = Add(x=9, y=w3877) -> (x+y=w3870:i32)
                          n1830 = Add(x=w3877, y=10) -> (x+y=w3868:i32)
                          n1831 = local read "csv作成表"() -> (w3864:string[][])
                          n1832 = Unbundle By Name(w3875) -> ("実測値(MAX)"=w3871:string, "実測値(MIN)"=w3872:string)
                          n1833 = Replace Array Subset(array=w3864, new element #1=w3871, index (row) #1=w3869, index (col) #1=w3870, new element #2=w3872, index (row) #2=w3869, index (col) #2=w3868) -> (w3866:string[][])
                          n1834 = Select(t=w3866, s=w3876, f=w3864) -> (s? t:f=w3867:string[][])
                          n1835 = local write "csv作成表"(w3867) -> ()
                        }
                        frame 8 {
                          w3887 = 2
                          # "B"
                          # "A"
                          # "csv作成の為表へクラスタ(実測値)書き込み"
                          # "⑤"
                          # "③"
                          # "④"
                          n1836 = local read "メインON/OFF_\n設定 9"() -> (w3898:T1)
                          n1837 = Unbundle By Name(w3898) -> ("使用ON/OFF"=w3894:bool)
                          n1838 = control-ref of="前回値転記用配列"() -> (w3892:refnum<vi>)
                          n1839 = local read "メイン設定_設定 9"() -> (w3899:T2)
                          n1840 = call "メイン_測定値配列_CSV転記サブ.vi"("メイン設定_設定入力"=w3899, "ループ反復数値入力"=w3896, "実測設定項目"=w3897, "使用ON/OFF"=w3894, "前回値転記用配列"=w3892) -> ("ループ反復数値出力"=w3895:i32, "メイン設定_設定出力"=w3893:T2)  [unwired: 5 in]
                          n1841 = local write "メイン設定_設定 9"(w3893) -> ()
                          n1842 = Add(x=10, y=w3895) -> (x+y=w3888:i32)
                          n1843 = Add(x=w3895, y=11) -> (x+y=w3886:i32)
                          n1844 = local read "csv作成表"() -> (w3882:string[][])
                          n1845 = Unbundle By Name(w3893) -> ("実測値(MAX)"=w3889:string, "実測値(MIN)"=w3890:string)
                          n1846 = Replace Array Subset(array=w3882, new element #1=w3889, index (row) #1=w3887, index (col) #1=w3888, new element #2=w3890, index (row) #2=w3887, index (col) #2=w3886) -> (w3884:string[][])
                          n1847 = Select(t=w3884, s=w3894, f=w3882) -> (s? t:f=w3885:string[][])
                          n1848 = local write "csv作成表"(w3885) -> ()
                        }
                        frame 9 {
                          w3905 = 2
                          # "B"
                          # "A"
                          # "csv作成の為表へクラスタ(実測値)書き込み"
                          # "⑤"
                          # "③"
                          # "④"
                          n1849 = local read "メインON/OFF_\n設定 10"() -> (w3916:T1)
                          n1850 = Unbundle By Name(w3916) -> ("使用ON/OFF"=w3912:bool)
                          n1851 = control-ref of="前回値転記用配列"() -> (w3910:refnum<vi>)
                          n1852 = local read "メイン設定_設定 10"() -> (w3917:T2)
                          n1853 = call "メイン_測定値配列_CSV転記サブ.vi"("メイン設定_設定入力"=w3917, "ループ反復数値入力"=w3914, "実測設定項目"=w3915, "使用ON/OFF"=w3912, "前回値転記用配列"=w3910) -> ("ループ反復数値出力"=w3913:i32, "メイン設定_設定出力"=w3911:T2)  [unwired: 5 in]
                          n1854 = local write "メイン設定_設定 10"(w3911) -> ()
                          n1855 = Add(x=11, y=w3913) -> (x+y=w3906:i32)
                          n1856 = Add(x=w3913, y=12) -> (x+y=w3904:i32)
                          n1857 = local read "csv作成表"() -> (w3900:string[][])
                          n1858 = Unbundle By Name(w3911) -> ("実測値(MAX)"=w3907:string, "実測値(MIN)"=w3908:string)
                          n1859 = Replace Array Subset(array=w3900, new element #1=w3907, index (row) #1=w3905, index (col) #1=w3906, new element #2=w3908, index (row) #2=w3905, index (col) #2=w3904) -> (w3902:string[][])
                          n1860 = Select(t=w3902, s=w3912, f=w3900) -> (s? t:f=w3903:string[][])
                          n1861 = local write "csv作成表"(w3903) -> ()
                        }
                        frame 10 {
                          w3923 = 2
                          # "B"
                          # "A"
                          # "csv作成の為表へクラスタ(実測値)書き込み"
                          # "⑤"
                          # "③"
                          # "④"
                          n1862 = local read "メインON/OFF_\n設定 11"() -> (w3934:T1)
                          n1863 = Unbundle By Name(w3934) -> ("使用ON/OFF"=w3930:bool)
                          n1864 = control-ref of="前回値転記用配列"() -> (w3928:refnum<vi>)
                          n1865 = local read "メイン設定_設定 11"() -> (w3935:T2)
                          n1866 = call "メイン_測定値配列_CSV転記サブ.vi"("メイン設定_設定入力"=w3935, "ループ反復数値入力"=w3932, "実測設定項目"=w3933, "使用ON/OFF"=w3930, "前回値転記用配列"=w3928) -> ("ループ反復数値出力"=w3931:i32, "メイン設定_設定出力"=w3929:T2)  [unwired: 5 in]
                          n1867 = local write "メイン設定_設定 11"(w3929) -> ()
                          n1868 = Add(x=12, y=w3931) -> (x+y=w3924:i32)
                          n1869 = Add(x=w3931, y=13) -> (x+y=w3922:i32)
                          n1870 = local read "csv作成表"() -> (w3918:string[][])
                          n1871 = Unbundle By Name(w3929) -> ("実測値(MAX)"=w3925:string, "実測値(MIN)"=w3926:string)
                          n1872 = Replace Array Subset(array=w3918, new element #1=w3925, index (row) #1=w3923, index (col) #1=w3924, new element #2=w3926, index (row) #2=w3923, index (col) #2=w3922) -> (w3920:string[][])
                          n1873 = Select(t=w3920, s=w3930, f=w3918) -> (s? t:f=w3921:string[][])
                          n1874 = local write "csv作成表"(w3921) -> ()
                        }
                        frame 11 {
                          w3941 = 2
                          # "B"
                          # "A"
                          # "csv作成の為表へクラスタ(実測値)書き込み"
                          # "⑤"
                          # "③"
                          # "④"
                          n1875 = local read "メインON/OFF_\n設定 12"() -> (w3952:T1)
                          n1876 = Unbundle By Name(w3952) -> ("使用ON/OFF"=w3948:bool)
                          n1877 = control-ref of="前回値転記用配列"() -> (w3946:refnum<vi>)
                          n1878 = local read "メイン設定_設定 12"() -> (w3953:T2)
                          n1879 = call "メイン_測定値配列_CSV転記サブ.vi"("メイン設定_設定入力"=w3953, "ループ反復数値入力"=w3950, "実測設定項目"=w3951, "使用ON/OFF"=w3948, "前回値転記用配列"=w3946) -> ("ループ反復数値出力"=w3949:i32, "メイン設定_設定出力"=w3947:T2)  [unwired: 5 in]
                          n1880 = local write "メイン設定_設定 12"(w3947) -> ()
                          n1881 = Add(x=13, y=w3949) -> (x+y=w3942:i32)
                          n1882 = Add(x=w3949, y=14) -> (x+y=w3940:i32)
                          n1883 = local read "csv作成表"() -> (w3936:string[][])
                          n1884 = Unbundle By Name(w3947) -> ("実測値(MAX)"=w3943:string, "実測値(MIN)"=w3944:string)
                          n1885 = Replace Array Subset(array=w3936, new element #1=w3943, index (row) #1=w3941, index (col) #1=w3942, new element #2=w3944, index (row) #2=w3941, index (col) #2=w3940) -> (w3938:string[][])
                          n1886 = Select(t=w3938, s=w3948, f=w3936) -> (s? t:f=w3939:string[][])
                          n1887 = local write "csv作成表"(w3939) -> ()
                        }
                      }
                    }
                  }
                }
                n1888 = local write "値転記用配列"(w3711) -> ()
                n1889 = flat-sequence {
